vi "Find Outlines.vi"(11 "Image Pixels (U8)":u8[][](array[numeric])) -> (1 "Mask out":i8[][](array[numeric]), 2 "Largest Outline":refnum<class "Outline.lvclass">)   [LabVIEW 2013]
uses:
  Outline/Outline.lvclass
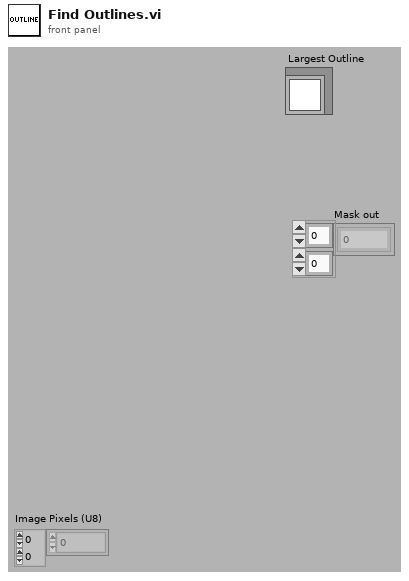
[diagram p1: front panel]
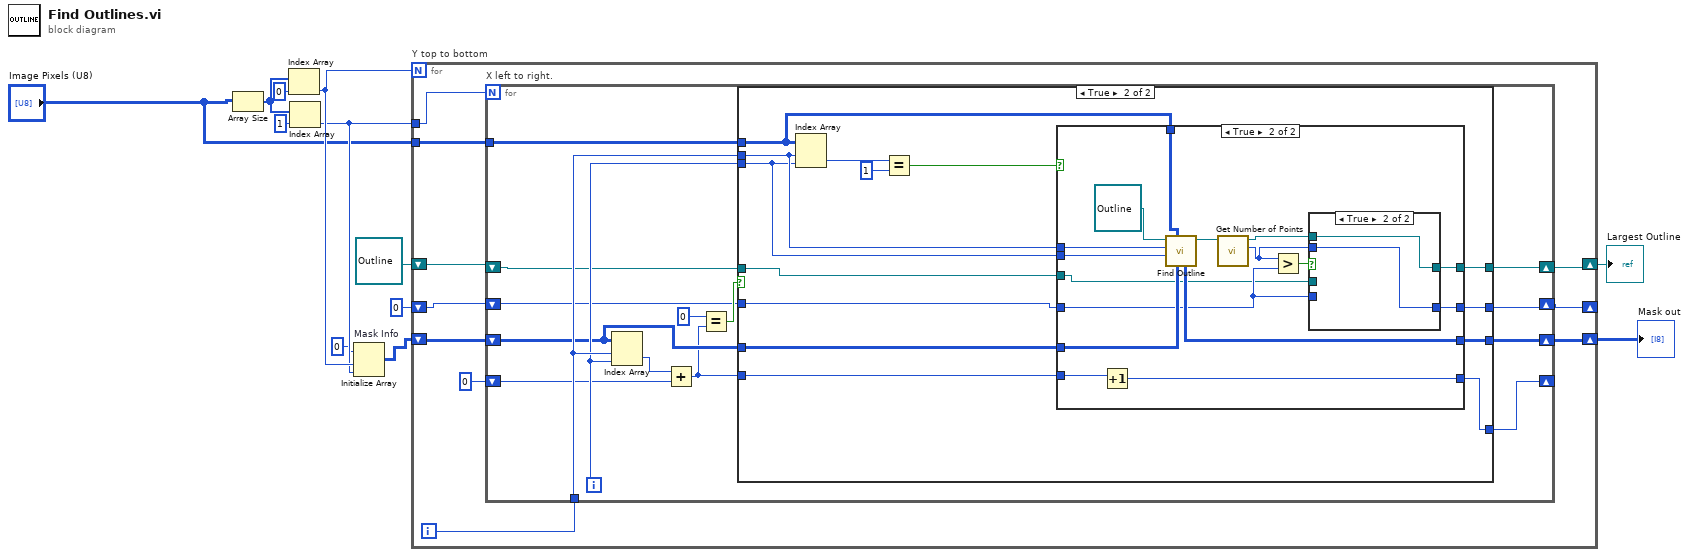
[diagram p0: block diagram]
diagram:
  n1 = Array Size(array="Image Pixels (U8)") -> (size(s)=w12:i32[])
  n2 = Index Array(array=w12, index=0) -> (element=w10:i32)
  n3 = Index Array(array=w12, index=1) -> (element=w9:i32)
  n4 = Initialize Array "Mask Info"(i8 0 ("index"), w10, w9) -> (w5:i8[][])
  n5 = for "Y top to bottom" {
    N: w10 -> [_]
    tunnel: w9 -> [w21]
    tunnel: "Image Pixels (U8)" -> [w20]
    shift-right: [w18] -> w4
    shift-left: w5 -> [w19]
    shift-right: [w15] -> w1
    shift-left: refnum<class "Outline.lvclass"> refnum ("Outline in") -> [w16]
    shift-right: [w13] -> _
    shift-left: 0 ("Number of points") -> [w14]
    i -> [w22]
    n6 = for "X left to right." {
      N: w21 -> [_]
      tunnel: w22 -> [w37]
      tunnel: w20 -> [w35]
      shift-right: [w30] -> w18
      shift-left: w19 -> [w31]
      shift-right: [w27] -> _
      shift-left: i8 0 ("index") -> [w28]
      shift-right: [w25] -> w15
      shift-left: w16 -> [w26]
      shift-right: [w23] -> w13
      shift-left: w14 -> [w24]
      i -> [w36]
      n7 = Index Array(array=w31, index (row)=w37, index (col)=w36) -> (element=w34:i8)
      n8 = Add(x=w34, y=w28) -> (x+y=w29:i8)
      n9 = Equal?(x=i8 0, y=w29) -> (x = y?=w32:bool)
      n10 = case shown="True" w32 {
        tunnel: w37 -> [_ w55]
        tunnel: w36 -> [_ w54]
        tunnel: w35 -> [_ w51]
        tunnel: w31 -> [w41 w53]
        tunnel: [w41 w52] -> w30
        tunnel: w29 -> [w40 w50]
        tunnel: [w40 w49] -> w27
        tunnel: w26 -> [w39 w48]
        tunnel: [w39 w47] -> w25
        tunnel: [w38 w43] -> w23
        tunnel: w24 -> [w38 w42]
        frame False {
        }
        frame True {
          n11 = Index Array(array=w51, index (row)=w55, index (col)=w54) -> (element=w46:u8)
          n12 = Equal?(x=w46, y=u8 1) -> (x = y?=w44:bool)
          n13 = case shown="True" w44 {
            tunnel: w55 -> [_ w75]
            tunnel: w54 -> [_ w74]
            tunnel: w53 -> [w59 w73]
            tunnel: [w59 w72] -> w52
            tunnel: w51 -> [_ w71]
            tunnel: w50 -> [w58 w70]
            tunnel: [w58 w69] -> w49
            tunnel: w48 -> [w57 w60]
            tunnel: [w57 w62] -> w47
            tunnel: [w56 w65] -> w43
            tunnel: w42 -> [w56 w63]
            frame False {
            }
            frame True {
              n14 = Increment(x=w70) -> (x+1=w69:i8)
              n15 = call-dynamic "Find Outline.vi"("Mask Info"=w73, "Data"=w71, "Starting X (left)"=w74, "Starting Y (top)"=w75, "Outline in"=refnum<class "Outline.lvclass"> refnum) -> ("Outline out"=w67:refnum<class "Outline.lvclass">, "Mask Info out"=w72:i8[][])  [unwired: 4 in, 1 out]
              n16 = call-dynamic "Get Number of Points.vi"("Outline in"=w67) -> ("Number of points"=w64:i32, "Outline out"=w61:refnum<class "Outline.lvclass">)  [unwired: 8 in, 1 out]
              n17 = Greater?(x=w64, y=w63) -> (0:w66:bool)
              n18 = case shown="True" w66 {
                tunnel: [w77 w79] -> w65
                tunnel: w64 -> [_ w79]
                tunnel: w63 -> [w77 _]
                tunnel: [w76 w78] -> w62
                tunnel: w61 -> [_ w78]
                tunnel: w60 -> [w76 _]
                frame False {
                }
                frame True {
                }
              }
            }
          }
        }
      }
    }
  }
  "Mask out" <- w4
  "Largest Outline" <- w1
